vi "Get Targets.vi"(8 "error in":errorcluster, 11 "Builder in":refnum<class "Builder.lvclass">) -> (0 "error out":errorcluster, 3 "Builder out":refnum<class "Builder.lvclass">)   [LabVIEW 2021, in "App-Builder Library.lvlib" / "Builder.lvclass"]
uses:
  Builder.lvclass
  Builder.lvclass/Builder.ctl
  Build specification.ctl
  App descriptions.ctl
  Build Type.ctl
panel:
  out "Current Version":string
  out "next version":string
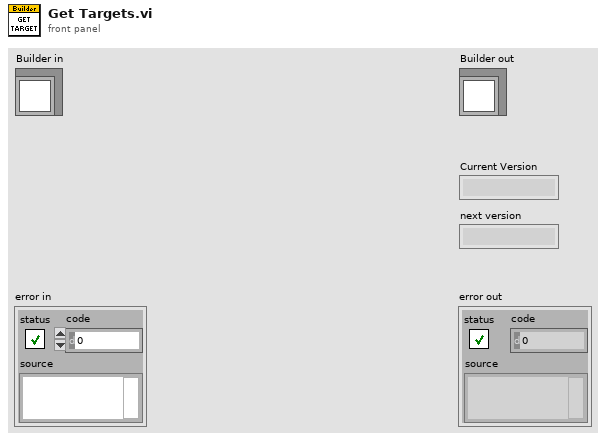
[diagram p1: front panel]
types:
  T1 = typedef "App-Builder Library.lvlib/Builder.lvclass/Build specification.ctl" = cluster{"target name":string, "Build specification":string, "Project Path":path}
  T2 = typedef "NI_App_Builder_API.lvlib/Build Specification Version.ctl" = cluster{"Major":u16, "Minor":u16, "Fix":u16, "Build":u16}
  T3 = typedef "App-Builder Library.lvlib/Builder.lvclass/App descriptions.ctl" = cluster{"App Name":string, "Build Type":T4, "Current Version":string, "Next Version":string, "Check":bool}
  T4 = typedef "App-Builder Library.lvlib/Builder.lvclass/Build Type.ctl" = enum16{"Major", "Minor", "Fix", "Build"}
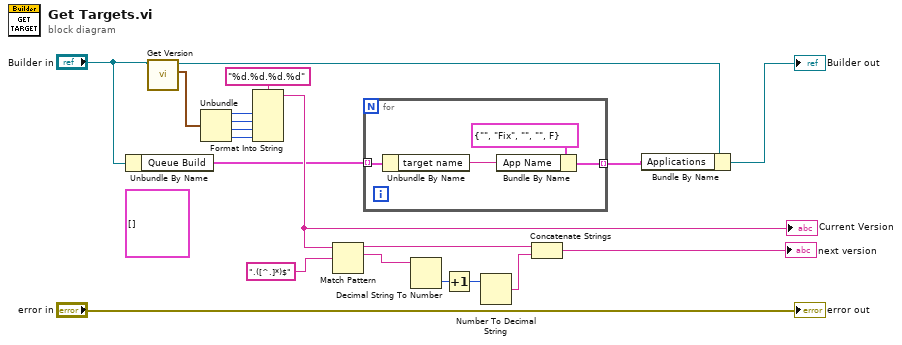
[diagram p0: block diagram]
diagram:
  (unwired) T1[] [] ("Queue Build")
  n1 = Unbundle By Name("Builder in") -> ("Queue Build"=w4:T1[])
  n2 = call-dynamic "Get Version.vi"("Builder in"="Builder in") -> ("Build Version"=w18:T2, "Builder out"=w3:refnum<class "Builder.lvclass">)  [unwired: 7 in, 2 out]
  n3 = Unbundle(w18) -> ("Major"=w14:u16, "Minor"=w15:u16, "Fix"=w16:u16, "Build"=w17:u16)
  n4 = Format Into String(format string="%d.%d.%d.%d", w14, w15, w16, w17) -> (resulting string=w12:string)  [unwired: 2 in, 1 out]
  "Current Version" <- w12
  n5 = Match Pattern(string=w12, regular expression=".([^.]*)$") -> (before substring=w10:string, match substring=w6:string)  [unwired: 1 in, 2 out]
  n6 = for {
    tunnel: [w23] -> w2 mode=indexing
    tunnel: w4 -> [w22] mode=indexing
    n7 = Unbundle By Name(w22) -> ("target name"=w21:string)
    n8 = Bundle By Name(cluster=T3 {"App Name"="", "Build Type"=enum."Fix", "Current Version"="", "Next Version"="", "Check"=FALSE} ("Applications"), "App Name"=w21) -> (w23:T3)
  }
  n9 = Decimal String To Number(string=w6) -> (number=w9:i32)  [unwired: 2 in, 1 out]
  n10 = Increment(x=w9) -> (x+1=w8:i32)
  n11 = Number To Decimal String(number=w8) -> (decimal integer string=w7:string)  [unwired: 1 in]
  n12 = Concatenate Strings(w10, w7) -> (→"next version":string)
  n13 = Bundle By Name(cluster=w3, "Applications"=w2) -> (→"Builder out":refnum<class "Builder.lvclass">)
  "error out" <- "error in"
